vi "WPILogBuildTree.vi"(8 "error in (no error)":errorcluster, 10 "Entity Tree":refnum<vi>, 11 "Data Value Reference in":refnum<data-value>) -> (0 "error out":errorcluster, 3 "Data Value Reference out":refnum<data-value>)   [LabVIEW 2020]
uses:
  Typedef/WPILibLog.ctl
  Typedef/Header.ctl
  Typedef/Entry.ctl
  Typedef/Record.ctl
  <vilib>/National Instruments/Tree Map/API/List Roots.vi
  <vilib>/National Instruments/Tree Map/Utility/Into Tree Control Items.vi
  <vilib>/National Instruments/Tree Map/Tree Map.lvlib
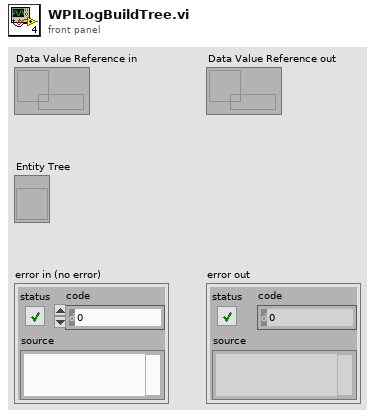
[diagram p1: front panel]
types:
  T1 = typedef "WPILibLog.ctl" = cluster{"Header":T2, "Record Start Idx":i32, "Entries":map{u32, T3}, "file ref":refnum<file>, "Finished Entries":T3[], "raw data":u8[]}
  T2 = typedef "Header.ctl" = cluster{"Header String":string, "Version":dbl, "Header Extra String Length":u32, "Header Extra String":string}
  T3 = typedef "Entry.ctl" = cluster{"ID":u32, "Records":T4[], "Finished?":bool, "Name":string, "Type":string, "Metadata":string, "RecordCnt":i32}
  T4 = typedef "Record.ctl" = cluster{"raw data":u8[], "ID":u32, "Size (bytes)":u32, "Timestamp":u64}
  T5 = typedef "Tree Map.lvlib/Tree Map Data.ctl" = map{string, cluster{"Child Paths Set":set{string}, "Name":string, "Data":string, "Attributes":map{string, string}}}
  T6 = cluster{"Left Cell String":string, "Child Text":string[], "Child Tag":string, "Item Indent":i32, "Child Only?":bool, "Glyph Index":i32}[]
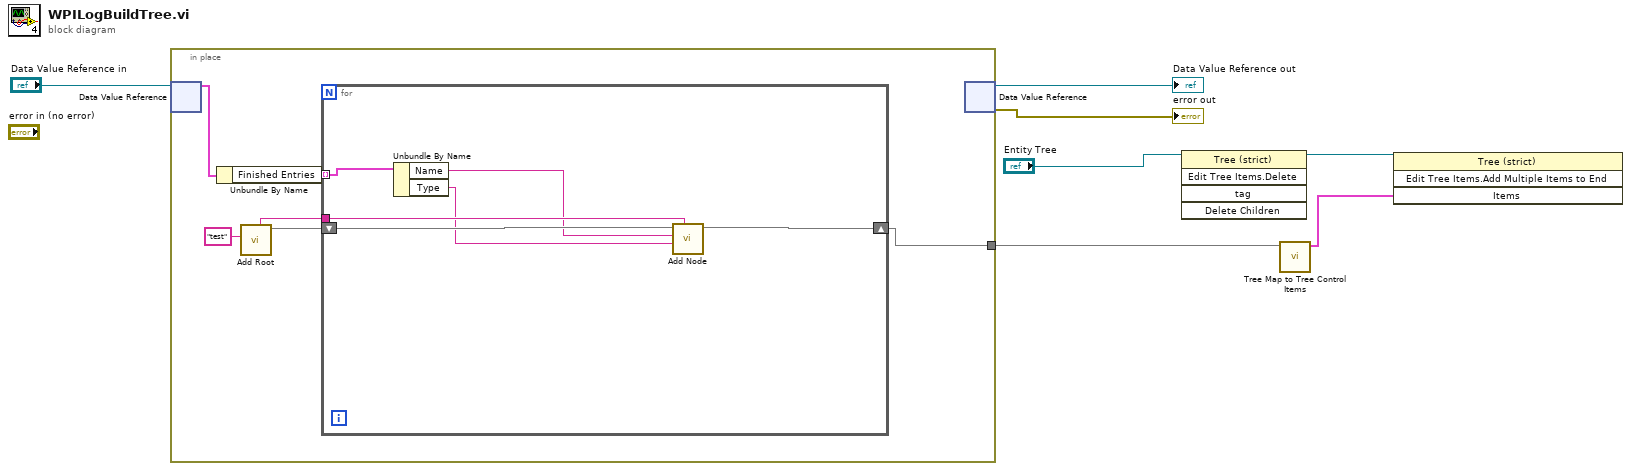
[diagram p0: block diagram]
diagram:
  n1 = in-place {
    in-place-border: [w8] -> w1
    n2 = in-place-dvr #1("Data Value Reference in") -> (w13:T1)  [unwired: 1 out]
    n3 = Unbundle By Name(w13) -> ("Finished Entries"=w12:T3[])
    n4 = call <vilib>:"Add Root.vi"("New Root Name"="test") -> ("Tree Map Out"=w10:T5, "Root Path"=w9:string)  [unwired: 9 in]
    n5 = for {
      tunnel: w12 -> [w16] mode=indexing
      tunnel: w9 -> [w18]
      shift-right: [w17] -> w8
      shift-left: w10 -> [w19]
      n6 = Unbundle By Name(w16) -> ("Name"=w15:string, "Type"=w14:string)
      n7 = call <vilib>:"Add Node.vi"("Parent Path"=w18, "Data"=w14, "New Node Name"=w15, "Tree Map In"=w19) -> ("Tree Map Out"=w17:T5)  [unwired: 5 in, 2 out]
    }
    n8 = in-place-dvr #1() -> (→"Data Value Reference out":refnum<data-value>, →"error out":errorcluster)  [unwired: 1 in]
  }
  n9 = invoke class="Tree (strict)" method="Edit Tree Items.Delete"(reference="Entity Tree") -> (reference out=w3:refnum<vi>)  [unwired: 4 in, 4 out]
  n10 = call <vilib>:"Tree Map to Tree Control Items.vi"("Tree Map In"=w1) -> ("Tree Control Items"=w2:T6)  [unwired: 10 in]
  n11 = invoke class="Tree (strict)" method="Edit Tree Items.Add Multiple Items to End"(reference=w3, "Items"=w2) -> ()  [unwired: 2 in, 4 out]
